vi "gun_rt_slow_downstream_datastore.vi"(10 "data_store_mode":enum16{"Set", "Get"}(ring), 11 "gun_rt_slow_downstream_data":T1) -> (3 "gun_rt_slow_downstream_data out":T1)   [LabVIEW 2011]
uses:
  gun_rt_slow_downstream_data.ctl
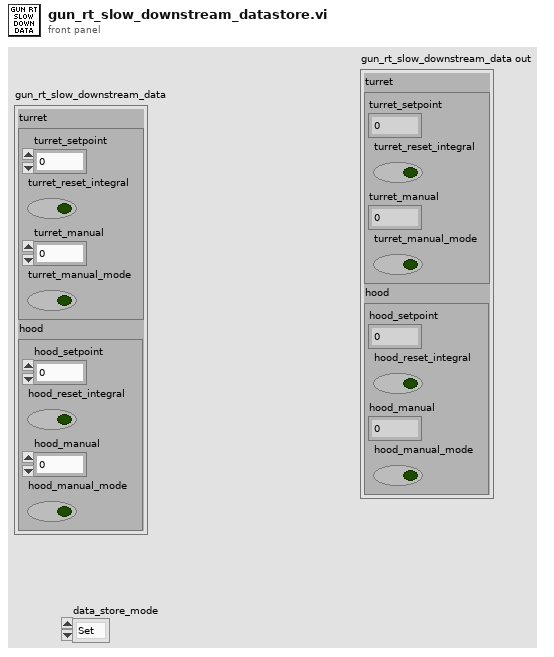
[diagram p1: front panel]
types:
  T1 = typedef "gun_rt_slow_downstream_data.ctl" = cluster{"turret":cluster{"turret_setpoint":dbl, "turret_reset_integral":bool, "turret_manual":dbl, "turret_manual_mode":bool}, "hood":cluster{"hood_setpoint":dbl, "hood_reset_integral":bool, "hood_manual":dbl, "hood_manual_mode":bool}}
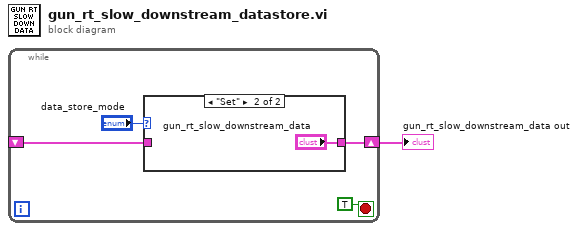
[diagram p0: block diagram]
diagram:
  n1 = while {
    shift-right: [w3] -> w1
    shift-left: _ -> [w2]
    stop <- TRUE stop-if-true
    n2 = case shown="\"Set\"" "data_store_mode" {
      tunnel: [w6 "gun_rt_slow_downstream_data"] -> w3
      tunnel: w2 -> [w6 _]
      frame "Get", Default {
      }
      frame "Set" {
      }
    }
  }
  "gun_rt_slow_downstream_data out" <- w1
